vi "CaptureImage.vi"(0 "Camera":T1="cam0", 1 "Rotate (degrees)":sgl, 2 "ImageName":string="name1", 5 "error in (no error)":errorcluster) -> (6 "Image":T2(plugin-control), 8 "error out":errorcluster)   [LabVIEW 2019]
uses:
  <vilib>/userDefined/High Color/IMAQdx.ctl
  <vilib>/vision/driver/NI_Vision_Acquisition_Software.lvlib
  <vilib>/vision/NI_Vision_Development_Module.lvlib
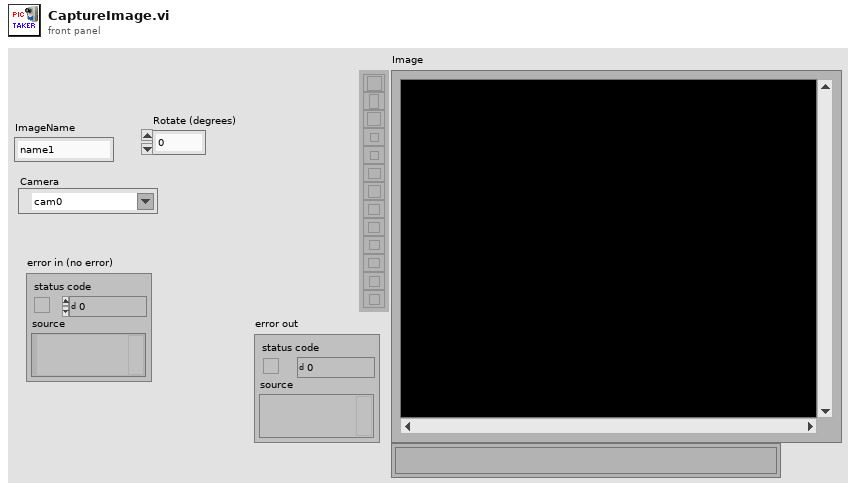
[diagram p1: front panel]
types:
  T1 = typedef "IMAQdx.ctl" = refnum<k21>
  T2 = typedef "IMAQ Image.ctl" = refnum<image>
  T3 = typedef "Image Type" = u32
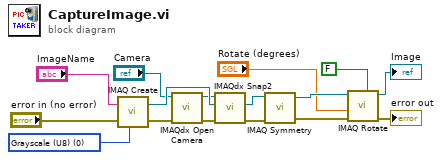
[diagram p0: block diagram]
diagram:
  w5 = T3 0 items=["Grayscale (U8)", "Grayscale (I16)", "Grayscale (SGL)", "Complex (CSG)", "RGB (U32)", "HSL (U32)", "RGB (U64)", "Grayscale (U16)"] ("Image Type")
  n1 = call "IMAQ Create"("Image Name"="ImageName", "Image Type"=w5, "error in (no error)"="error in (no error)") -> ("New Image"=w15:T2, "error out"=w13:errorcluster)  [unwired: 2 in]
  n2 = call <vilib>:"IMAQdx Open Camera.vi"("error in"=w13, "Session In"="Camera") -> ("error out"=w16:errorcluster, "Session Out"=w14:T1)  [unwired: 8 in]
  n3 = call <vilib>:"IMAQdx Snap2.vi"("error in"=w16, "Image In"=w15, "Session In"=w14) -> ("error out"=w8:errorcluster, "Image Out"=w9:T2)  [unwired: 6 in, 1 out]
  n4 = call "IMAQ Symmetry"("error in (no error)"=w8, "Image Src"=w9) -> ("error out"=w7:errorcluster, "Image Dst Out"=w12:T2)  [unwired: 3 in]
  n5 = call "IMAQ Rotate"("Maintain Size"=FALSE, "error in (no error)"=w7, "Angle (degrees)"="Rotate (degrees)", "Image Src"=w12) -> ("error out"=→"error out":errorcluster, "Image Dst Out"=→"Image":T2)  [unwired: 6 in]
